vi "Parse Multiline Basic String.vi"(8 "error in (no error)":errorcluster, 10 "start at":i32, 11 "TOML String":string) -> (0 "error out":errorcluster, 2 "offset past match":i32, 3 "String":string)   [LabVIEW 2019, in "BlueTOMLSerializer.lvlib"]
uses:
  BlueTOMLSerializer.lvlib
  <vilib>/regexp/Match Regular Expression.xnode
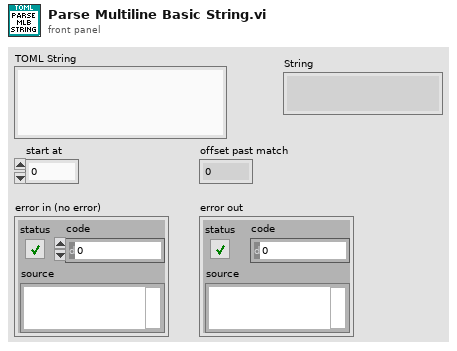
[diagram p1: front panel]
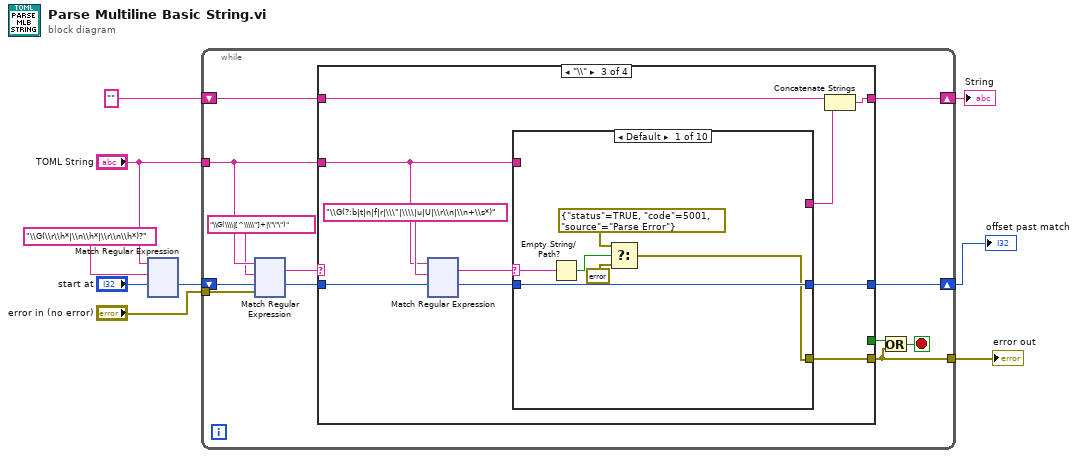
[diagram p0: block diagram]
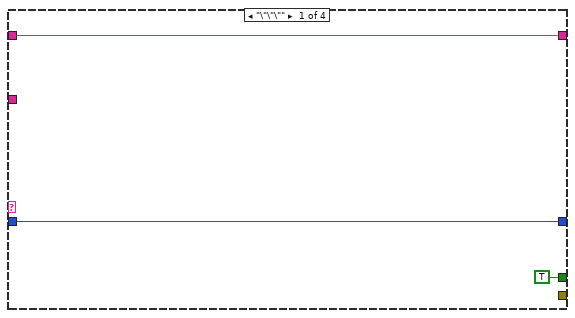
[diagram p2: hidden frame]
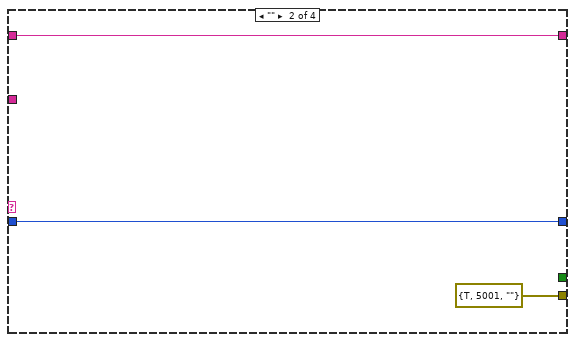
[diagram p3: hidden frame]
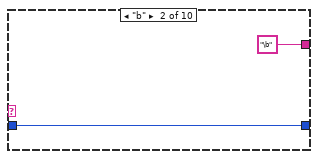
[diagram p4: hidden frame]
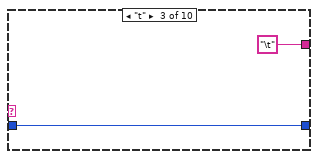
[diagram p5: hidden frame]
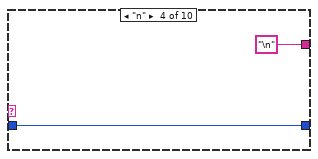
[diagram p6: hidden frame]
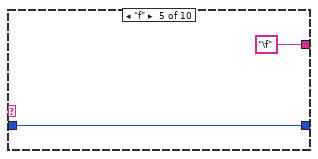
[diagram p7: hidden frame]
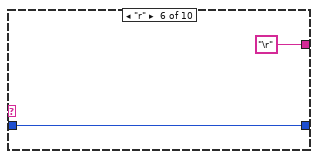
[diagram p8: hidden frame]
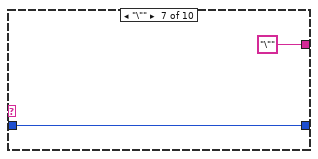
[diagram p9: hidden frame]
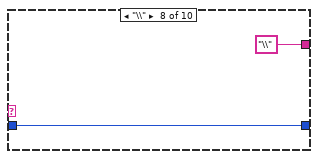
[diagram p10: hidden frame]
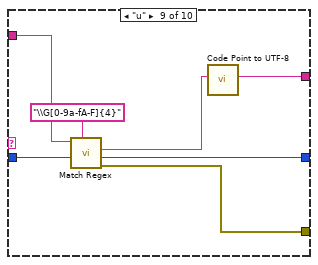
[diagram p11: hidden frame]
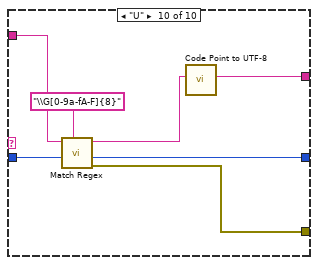
[diagram p12: hidden frame]
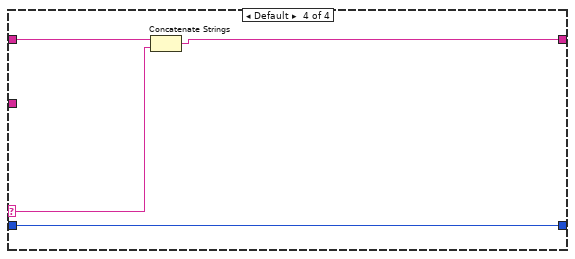
[diagram p13: hidden frame]
diagram:
  n1 = xnode "Match Regular Expression"("input string"="TOML String", "regular expression"="\\G(\\r\\h*|\\n\\h*|\\r\\n\\h*)?", "offset (0)"="start at") -> ("offset past match"=w3:i32)  [unwired: 3 in, 4 out]
  n2 = while {
    tunnel: "error in (no error)" -> [w21]
    tunnel: "TOML String" -> [w14]
    shift-right: [w19] -> w5
    shift-left: w3 -> [w20]
    shift-right: [w17] -> w6
    shift-left: "" -> [w16]
    tunnel: [w12] -> w7
    stop <- w13 stop-if-true
    n3 = xnode "Match Regular Expression"("input string"=w14, "regular expression"="\\G(\\\\|[^\\\\\"]+|\"\"\")", "offset (0)"=w20, "error in"=w21) -> ("whole match"=w11:string, "offset past match"=w18:i32)  [unwired: 2 in, 3 out]
    n4 = case shown="\"\\\\\"" w11 {
      selector: w11 -> [_ _ _ w188]
      tunnel: [w23 w26 w33 w189] -> w19
      tunnel: w18 -> [w23 w26 w36 w189]
      tunnel: [w24 w27 w31 w186] -> w17
      tunnel: w16 -> [w24 w27 w37 w187]
      tunnel: [TRUE _ _ _] -> w15
      tunnel: w14 -> [_ _ w29 _]
      tunnel: [_ errorcluster {"status"=TRUE, "code"=5001, "source"=""} ("error constant") w34 _] -> w12
      frame "\"\"\"" {
      }
      frame "" {
      }
      frame "\\" {
        n5 = xnode "Match Regular Expression"("input string"=w29, "regular expression"="\\G(?:b|t|n|f|r|\\\"|\\\\|u|U|\\r\\n|\\n+\\s*)", "offset (0)"=w36) -> ("whole match"=w28:string, "offset past match"=w32:i32)  [unwired: 3 in, 3 out]
        n6 = case shown="Default" w28 {
          selector: w28 -> [w42 _ _ _ _ _ _ _ _ _]
          tunnel: [w38 _ _ _ _ _ _ _ w61 w67] -> w34
          tunnel: [w43 w44 w46 w48 w50 w52 w54 w56 w62 w68] -> w33
          tunnel: w32 -> [w43 w44 w46 w48 w50 w52 w54 w56 w63 w69]
          tunnel: [_ "\b" ("regular expression") "\t" ("regular expression") "\n" ("regular expression") "\f" ("regular expression") "\r" ("regular expression") "\"" ("regular expression") "\\" ("regular expression") w58 w65] -> w30
          tunnel: w29 -> [_ _ _ _ _ _ _ _ w64 w70]
          frame Default {
            n7 = Empty String/Path?(string/path=w42) -> (empty?=w41:bool)
            n8 = Select(t=errorcluster {"status"=TRUE, "code"=5001, "source"="Parse Error"} ("error constant"), s=w41, f=errorcluster {"status"=FALSE, "code"=0, "source"=""}) -> (s? t:f=w38:errorcluster)
          }
          frame "b" {
          }
          frame "t" {
          }
          frame "n" {
          }
          frame "f" {
          }
          frame "r" {
          }
          frame "\"" {
          }
          frame "\\" {
          }
          frame "u" {
            n9 = call "Match Regex.vi"("regular expression"="\\G[0-9a-fA-F]{4}", "offset"=w63, "String"=w64) -> ("error out"=w61:errorcluster, "offset past match"=w62:i32, "submatch 1"=w59:string)  [unwired: 5 in, 1 out]
            n10 = call "Code Point to UTF-8.vi"("Code Point"=w59) -> ("UTF-8"=w58:string)  [unwired: 10 in]
          }
          frame "U" {
            n11 = call "Match Regex.vi"("regular expression"="\\G[0-9a-fA-F]{8}", "offset"=w69, "String"=w70) -> ("error out"=w67:errorcluster, "offset past match"=w68:i32, "whole match"=w66:string)  [unwired: 5 in, 1 out]
            n12 = call "Code Point to UTF-8.vi"("Code Point"=w66) -> ("UTF-8"=w65:string)  [unwired: 10 in]
          }
        }
        n13 = Concatenate Strings(w37, w30) -> (w31:string)
      }
      frame Default {
        n14 = Concatenate Strings(w187, w188) -> (w186:string)
      }
    }
    n15 = Or(x=w15, y=w12) -> (x .or. y?=w13:bool)
  }
  "error out" <- w7
  "offset past match" <- w5
  "String" <- w6
